vi "RS_Remap.vi"(0 "appended path":path, 1 "mod_data":cdb[](array[numeric]), 2 "rs_slot1":cdb[](array[numeric]), 3 "rs_slot2":cdb[](array[numeric]), 4 "error in (no error)":errorcluster caption="错误输入（无错误）", 5 "prb_num":dbl, 7 "rbstart":dbl) -> (6 "remapdata":cdb[][](array[numeric]), 8 "error IO":errorcluster)   [LabVIEW 2015]
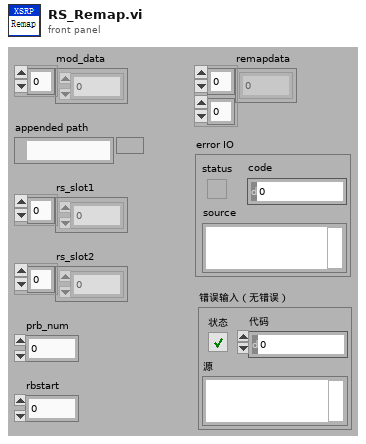
[diagram p1: front panel]
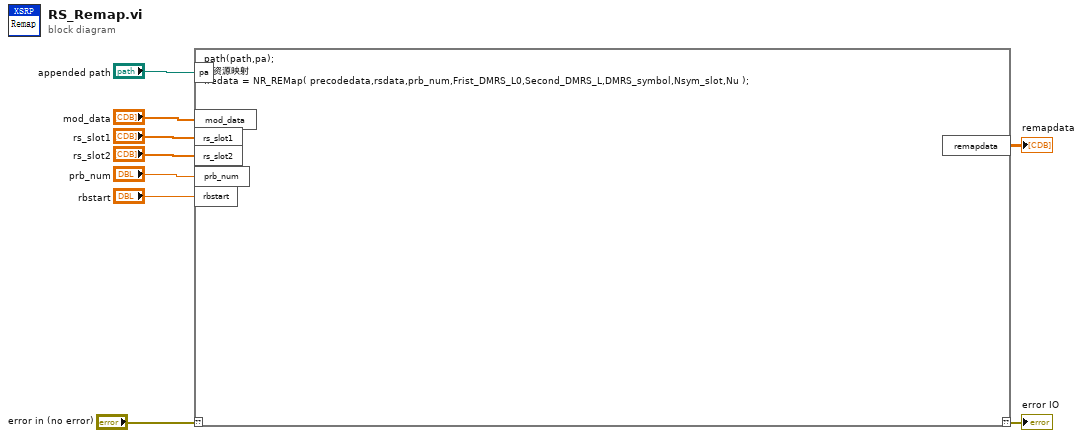
[diagram p0: block diagram]
diagram:
  n1 = script code="path(path,pa);\n%资源映射\nfredata = NR_REMap( precodedata,rsdata,prb_num,Frist_DMRS_L0,Second_DMRS_L,DMRS_symbol,Nsym_slot,Nu );"("??"="error in (no error)", "pa"="appended path", "mod_data"="mod_data", "rs_slot1"="rs_slot1", "rs_slot2"="rs_slot2", "prb_num"="prb_num", "rbstart"="rbstart") -> ("??"=→"error IO":errorcluster, "remapdata"=→"remapdata":cdb[][])
